vi "parseReadBoosterValveGainResponse.vi"(8 "error in (no error)":errorcluster, 10 "DynamicFrameParser":refnum<class "DynamicFrameParser.lvclass">, 11 "FAILC in":refnum<class "FAILC.lvclass">) -> (0 "error out":errorcluster, 3 "FAILC out":refnum<class "FAILC.lvclass">)   [LabVIEW 2016, in "RTFAILC.lvlib" / "FAILC.lvclass"]
uses:
  FAILC.lvclass
  Common_RT_Modbus/DynamicFrameParser/DynamicFrameParser.lvclass
  Common_RT_Modbus/DataTypes/ExceptionCodes.ctl
  FAILC.lvclass/FAILC.ctl
  Common_RT_Modbus/RTModbus.lvlib
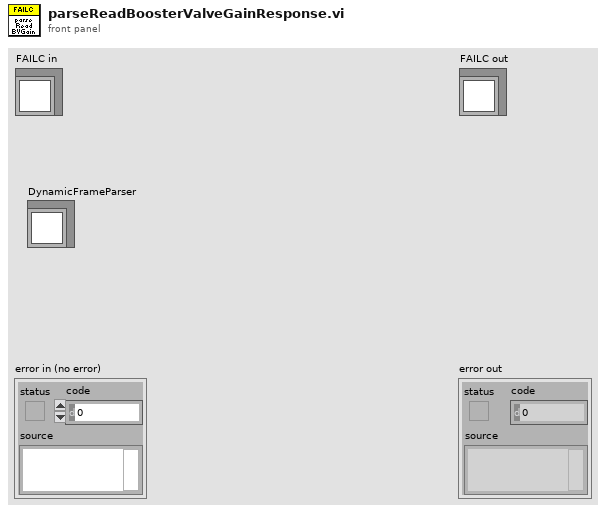
[diagram p1: front panel]
types:
  T1 = typedef "RTModbus.lvlib/ExceptionCodes.ctl" = u16
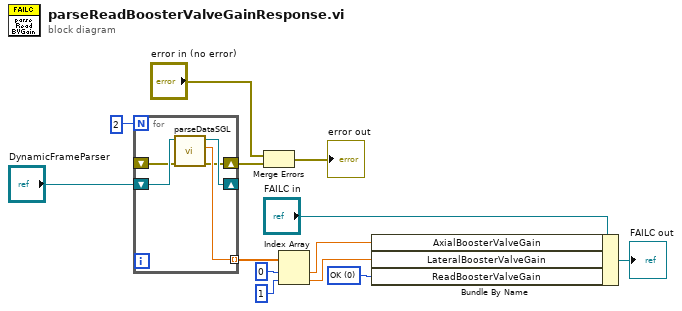
[diagram p0: block diagram]
diagram:
  w2 = T1 0 items=["OK", "IllegalFunction", "IllegalDataAddress", "IllegalDataValue", "SlaveDeviceFailure", "Acknowledge", "SlaveDeviceBusy", "NegativeAcknowledge", "MemoryParityError", "GatewayPathUnavailable", "GatewayTargetDeviceFailedToRespond"] ("FAData.FAResponses.PIDParameters")
  n1 = for {
    N: 2 -> [_]
    shift-right: [w17] -> _
    shift-left: "DynamicFrameParser" -> [w18]
    tunnel: [w16] -> w10 mode=indexing
    shift-right: [w14] -> w5
    shift-left: _ -> [w15]
    n2 = call "parseDataSGL.vi"("error in (no error)"=w15, "FrameParser in"=w18) -> ("error out"=w14:errorcluster, "Data"=w16:sgl, "FrameParser out"=w17:refnum<class "DynamicFrameParser.lvclass">)  [unwired: 7 in]
  }
  n3 = Merge Errors("error in (no error)", w5) -> (→"error out":errorcluster)
  n4 = Index Array(array=w10, index #1=0 ("index"), index #2=1 ("index")) -> (element #1=w7:sgl, element #2=w1:sgl)
  n5 = Bundle By Name(cluster="FAILC in", "AxialBoosterValveGain"=w7, "LateralBoosterValveGain"=w1, "ReadBoosterValveGain"=w2) -> (→"FAILC out":refnum<class "FAILC.lvclass">)
